vi "Write PWM Line.vi"(7 "PWM line":T1=1700 items=["Port0/DIO4 (Left Motor)"=1004, "Port0/DIO5 (Right Motor)"=1005, "Port0/DIO7 (Servo)"=1007, "Port7/DIO0"=1700, "Port7/DIO1"=1701, "Port7/DIO2"=1702, "Port7/DIO3"=1703], 8 "error in (no error)":errorcluster, 9 "pulse width (us)":u32=1500, 10 "period (us)":u32=20000, 11 "starter kit host in":refnum<class "NI_Robotics_Starter Kit Host.lvclass">) -> (0 "error out":errorcluster, 3 "starter kit host out":refnum<class "NI_Robotics_Starter Kit Host.lvclass">)   [LabVIEW 2017, in "NI_Robotics_Starter Kit Host.lvclass"]
doc: "Generates a pulse width modulation (PWM) output on a digital I/O line of the Starter Kit FPGA."
uses:
  <vilib>/robotics/Starter Kit/Host Interface/NI_Robotics_Starter Kit Host.lvclass
  <vilib>/robotics/Starter Kit/Direct IO/PWM Lines.ctl
  <vilib>/robotics/Starter Kit/Host Interface/NI_Robotics_Starter Kit Host.lvclass/NI_Robotics_Starter Kit Host.ctl
  <vilib>/robotics/Utilities/Generate Error.vi
  <vilib>/robotics/Starter Kit/Direct IO/NI_Robotics_Starter Kit Direct IO.lvclass
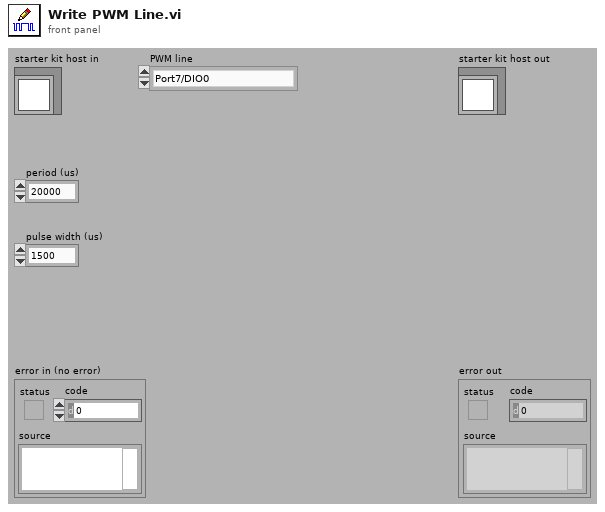
[diagram p1: front panel]
types:
  T1 = typedef "NI_Robotics_Starter Kit Direct IO.lvclass/PWM Lines.ctl" = u16
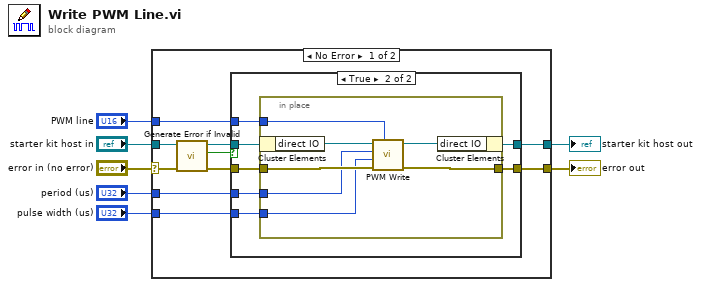
[diagram p0: block diagram]
diagram:
  n1 = case shown="No Error" "error in (no error)" {
    selector: "error in (no error)" -> [w10 w35]
    tunnel: [w15 w35] -> w6
    tunnel: [w17 w34] -> w4
    tunnel: "starter kit host in" -> [w12 w34]
    tunnel: "PWM line" -> [w16 _]
    tunnel: "period (us)" -> [w14 _]
    tunnel: "pulse width (us)" -> [w13 _]
    frame No Error {
      n2 = call <vilib>:"Generate Error if Invalid.vi"("error in (no error)"=w10, "starter kit host in"=w12) -> ("error out"=w9:errorcluster, "valid?"=w8:bool, "starter kit host out"=w11:refnum<class "NI_Robotics_Starter Kit Host.lvclass">)  [unwired: 7 in]
      n3 = case shown="True" w8 {
        tunnel: [w19 w26] -> w17
        tunnel: w16 -> [_ w25]
        tunnel: [w18 w24] -> w15
        tunnel: w14 -> [_ w23]
        tunnel: w13 -> [_ w22]
        tunnel: w11 -> [w19 w21]
        tunnel: w9 -> [w18 w20]
        frame False {
        }
        frame True {
          n4 = in-place {
            in-place-border: w25 -> [w31]
            in-place-border: w20 -> [w30]
            in-place-border: [w29] -> w24
            in-place-border: w23 -> [w28]
            in-place-border: w22 -> [w27]
            n5 = in-place-cluster #1(w21) -> ("direct IO"=w33:refnum<class "NI_Robotics_Starter Kit Direct IO.lvclass">)
            n6 = call-dynamic "PWM Write.vi"("PWM line"=w31, "error in (no error)"=w30, "pulse width (us)"=w27, "period (us)"=w28, "direct IO in"=w33) -> ("error out"=w29:errorcluster, "direct IO out"=w32:refnum<class "NI_Robotics_Starter Kit Direct IO.lvclass">)  [unwired: 5 in]
            n7 = in-place-cluster #1("direct IO"=w32) -> (w26:refnum<class "NI_Robotics_Starter Kit Host.lvclass">)
          }
        }
      }
    }
    frame Error {
    }
  }
  "error out" <- w6
  "starter kit host out" <- w4
